vi "Close Transport.vi"(8 "error in (no error)":errorcluster, 11 "StreamToDiskTransport":refnum<class "StreamToDiskTransport.lvclass">) -> (0 "error out":errorcluster)   [LabVIEW 2018, in "MVA Framework.lvlib" / "StreamToDiskTransport.lvclass"]
doc: "关闭传输"
uses:
  StreamToDiskTransport.lvclass
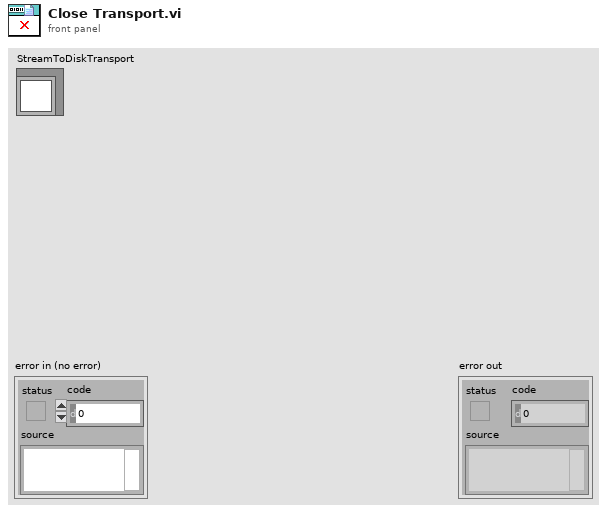
[diagram p1: front panel]
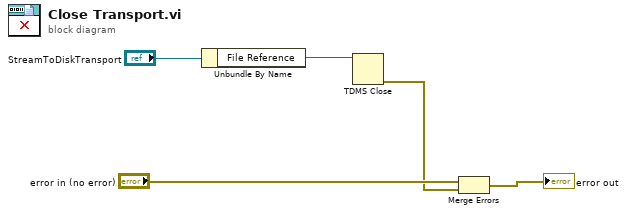
[diagram p0: block diagram]
diagram:
  n1 = Unbundle By Name("StreamToDiskTransport") -> ("File Reference"=w3:refnum<k34>)
  n2 = TDMS Close(11:w3) -> (0:w1:errorcluster)  [unwired: 1 in, 1 out]
  n3 = Merge Errors("error in (no error)", w1) -> (→"error out":errorcluster)
